vi "onTestDiscovery.vi"(8 "error in (no error)":errorcluster, 11 "Test Runner.Library in":refnum<class "Test Runner.Library.lvclass">) -> (0 "error out":errorcluster, 2 "Tests VIs":path[](array[path]), 3 "Test Runner.Library out":refnum<class "Test Runner.Library.lvclass">)   [LabVIEW 2013, in "Caraya.lvlib" / "Test Runner.Library.lvclass"]
uses:
  Test Runner.Library.lvclass
  Test Runner.Library.lvclass/Test Runner.Library.ctl
  Test/Define Test.vi
  Test/Test.lvclass
  Test Runner/Test Runner.lvclass
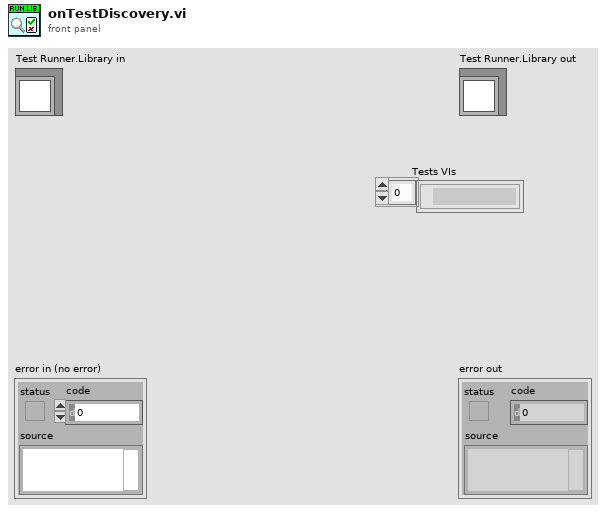
[diagram p1: front panel]
types:
  T1 = typedef "NI_FileType.lvlib/LVFileType.ctl" = enum32{"Invalid file", "Unknown type", "Instrument", "Control", "Polymorphic VI", "Project", "Library", "LVClass", "XControl", "XNode", "Shared library", ".NET assembly", "ActiveX interface", "CIN", "Run-time menu", "Palette menu", "Help file", "LLB", "XNode Edit Dependency", "Class Private Data Control", "Statechart", "MathScript .m file", "Ladder Diagram", "LVLibp"}
  T2 = cluster{"path":path, "delimited name":string, "type":T1, "iState":u32, "iStyle":u16, "wStyle":u16, "buttons":u16, "viflags":u32, "viflags2":u32, "links":u32[]}[]
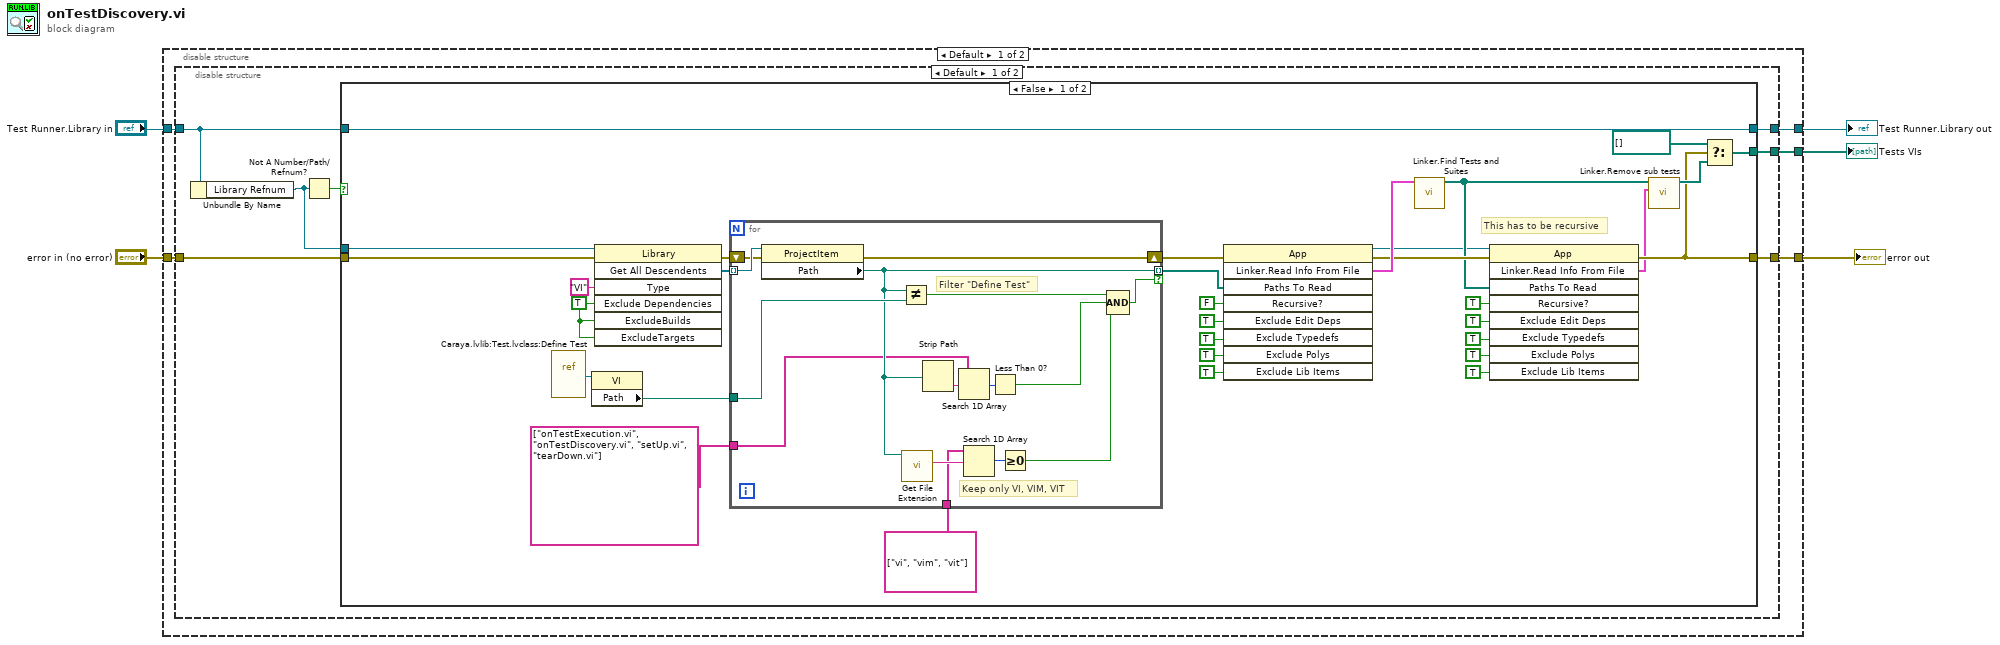
[diagram p0: block diagram]
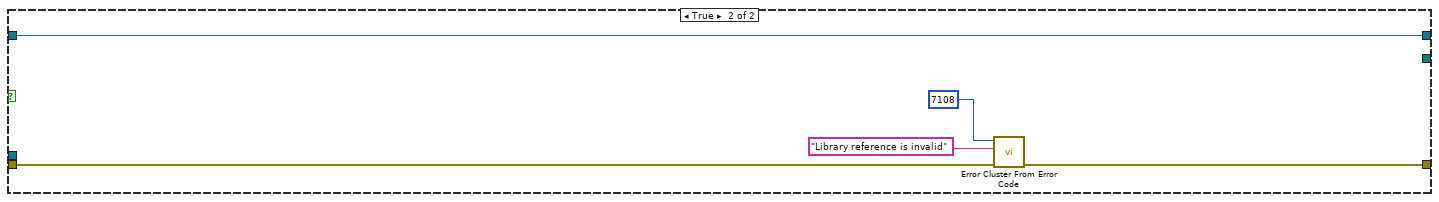
[diagram p2: hidden frame]
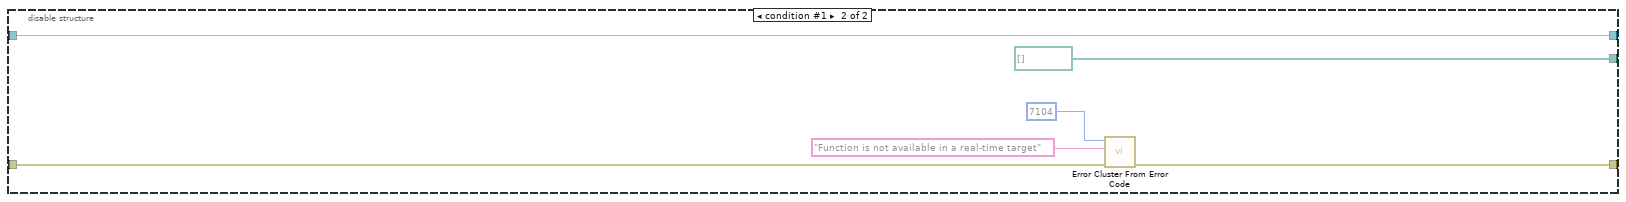
[diagram p3: hidden frame]
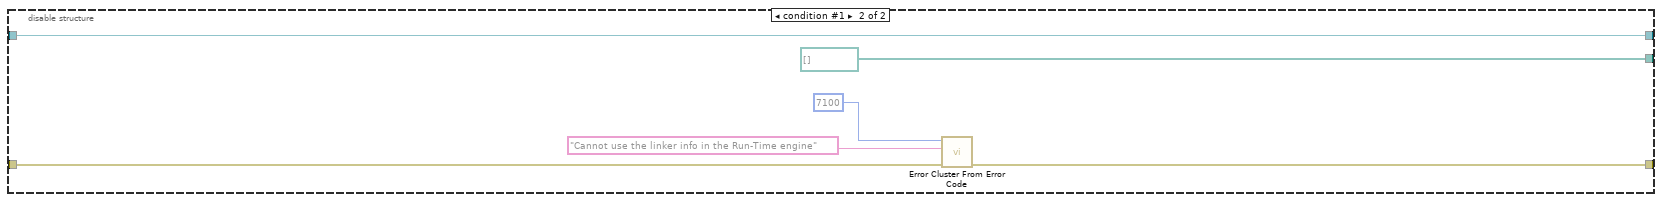
[diagram p4: hidden frame]
diagram:
  n1 = disable-structure shown="Default" {
    disable-tunnel: [w10 w79] -> w3
    disable-tunnel: "Test Runner.Library in" -> [w6 w78]
    disable-tunnel: [w9 w78] -> w1
    disable-tunnel: [w8 path[] [] ("Test VIs")] -> w2
    disable-tunnel: "error in (no error)" -> [w7 w76]
    frame condition #0 (active) {
      n2 = disable-structure shown="Default" {
        disable-tunnel: [w17 w71] -> w10
        disable-tunnel: [w16 w75] -> w9
        disable-tunnel: [w15 path[] [] ("Test VIs")] -> w8
        disable-tunnel: w7 -> [w13 w72]
        disable-tunnel: w6 -> [w12 w75]
        frame condition #0 (active) {
          n3 = Unbundle By Name(w12) -> ("Library Refnum"=w11:refnum<vi>)
          n4 = Not A Number/Path/Refnum?(number/path/refnum=w11) -> (NaN/Path/Refnum?=w14:bool)
          n5 = case shown="False" w14 {
            tunnel: [w24 w65] -> w17
            tunnel: [w44 _] -> w15
            tunnel: w11 -> [w18 _]
            tunnel: w12 -> [w32 w69]
            tunnel: [w32 w69] -> w16
            tunnel: w13 -> [w19 w66]
            frame False {
              w39 = TRUE ("ExcludeDependencies")
              # "This has to be recursive"
              n6 = vi-ref "Caraya.lvlib:Test.lvclass:Define Test.vi"() -> (w42:refnum<vi>)
              n7 = property class="VI"(reference=w42) -> ("Path"=w36:path)  [unwired: 1 in, 2 out]
              n8 = invoke class="Library" method="Get All Descendents"(reference=w18, error in=w19, "Type"="VI", "Exclude Dependencies"=w39, "ExcludeBuilds"=w39, "ExcludeTargets"=w39) -> (error out=w41:errorcluster, "All Descendents"=w40:refnum<vi>[])  [unwired: 1 in, 5 out]
              n9 = for {
                tunnel: w40 -> [w64] mode=indexing
                tunnel: [w54] -> w35 mode=indexing if=w58
                shift-right: [w62] -> w34
                shift-left: w41 -> [w63]
                tunnel: w36 -> [w61]
                tunnel: string[] ["vi", "vim", "vit"] -> [w56]
                tunnel: string[] ["onTestExecution.vi", "onTestDiscovery.vi", "setUp.vi", "tearDown.vi"] -> [w53]
                # "Keep only VI, VIM, VIT"
                # "Filter \"Define Test\""
                n10 = property class="ProjectItem"(reference=w64, error in=w63) -> (error out=w62:errorcluster, "Path"=w54:path)  [unwired: 1 out]
                n11 = Not Equal?(x=w54, y=w61) -> (x != y?=w59:bool)
                n12 = call <vilib>:"Get File Extension.vi"("file"=w54) -> ("lowercase file extension"=w57:string)  [unwired: 7 in, 3 out]
                n13 = Strip Path(path=w54) -> (name=w52:string)  [unwired: 1 out]
                n14 = Search 1D Array(1D array=w53, element=w52) -> (index of element=w51:i32)  [unwired: 1 in]
                n15 = Search 1D Array(1D array=w56, element=w57) -> (index of element=w60:i32)  [unwired: 1 in]
                n16 = Less Than 0?(x=w51) -> (x < 0?=w50:bool)
                n17 = Greater Or Equal To 0?(x=w60) -> (x >= 0?=w55:bool)
                n18 = Compound Arithmetic op=AND(w59, w50, w55) -> (w58:bool)
              }
              n19 = invoke class="App" method="Linker.Read Info From File"(error in=w34, "Paths To Read"=w35, "Recursive?"=FALSE, "Exclude Edit Deps"=TRUE ("Exclude Edit Time Dependencies"), "Exclude Typedefs"=TRUE, "Exclude Polys"=TRUE ("Exclude Poly VIs"), "Exclude Lib Items"=TRUE ("Exclude Unused Library Items")) -> (reference out=w20:refnum<vi>, error out=w25:errorcluster, "Linker.Read Info From File"=w37:T2)  [unwired: 2 in, 6 out]
              n20 = call "Linker.Find Tests and Suites.vi"("Linker:Read Info From File"=w37) -> ("All VIs defining a test (excluding those defining a suite)"=w22:path[])  [unwired: 8 in, 2 out]
              n21 = invoke class="App" method="Linker.Read Info From File"(reference=w20, error in=w25, "Paths To Read"=w22, "Recursive?"=TRUE, "Exclude Edit Deps"=TRUE ("Exclude Edit Time Dependencies"), "Exclude Typedefs"=TRUE, "Exclude Polys"=TRUE ("Exclude Poly VIs"), "Exclude Lib Items"=TRUE ("Exclude Unused Library Items")) -> (error out=w24:errorcluster, "Linker.Read Info From File"=w23:T2)  [unwired: 1 in, 7 out]
              n22 = call "Linker.Remove sub tests.vi"("Linker.Read Info From File"=w23, "Tests"=w22) -> ("Array"=w31:path[])  [unwired: 9 in]
              n23 = Select(t=path[] [], s=w24, f=w31) -> (s? t:f=w44:path[])
            }
            frame True {
              n24 = call <vilib>:"Error Cluster From Error Code.vi"("error in (no error)"=w66, "error message (\"\")"="Library reference is invalid" ("error message (\"\")"), "error code (0)"=7108) -> ("error out"=w65:errorcluster)  [unwired: 6 in]
            }
          }
        }
        frame condition #1 {
          n25 = call <vilib>:"Error Cluster From Error Code.vi"("error in (no error)"=w72, "error message (\"\")"="Function is not available in a real-time target" ("error message (\"\")"), "error code (0)"=7104) -> ("error out"=w71:errorcluster)  [unwired: 6 in]
        }
      }
    }
    frame condition #1 {
      n26 = call <vilib>:"Error Cluster From Error Code.vi"("error in (no error)"=w76, "error message (\"\")"="Cannot use the linker info in the Run-Time engine" ("error message (\"\")"), "error code (0)"=7100) -> ("error out"=w79:errorcluster)  [unwired: 6 in]
    }
  }
  "error out" <- w3
  "Test Runner.Library out" <- w1
  "Tests VIs" <- w2
